vi "make_filename.vi"(8 "error in (no error)":errorcluster, 10 "Storage parameters":T1, 11 "Fileno.":i32) -> (0 "error out":errorcluster, 3 "Path":path)   [LabVIEW 2010]
uses:
  typedefs/storage_parameters_cluster.ctl
panel:
  # "_0000.txt"
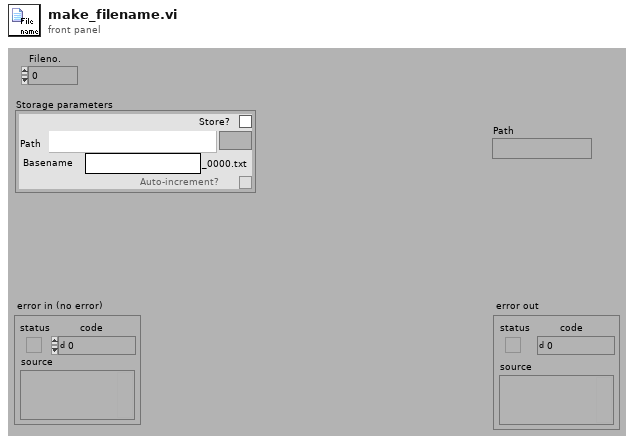
[diagram p1: front panel]
types:
  T1 = typedef "storage_parameters_cluster.ctl" = cluster{"Store?":bool, "Path":path, "Basename":string, "Auto-increment?":bool}
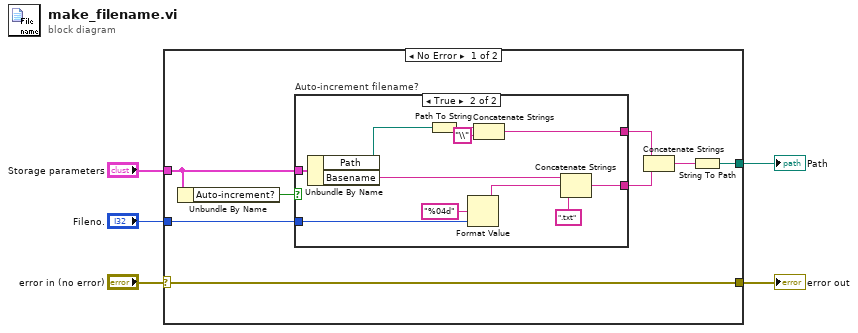
[diagram p0: block diagram]
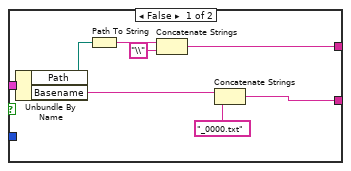
[diagram p2: hidden frame]
diagram:
  n1 = case shown="No Error" "error in (no error)" {
    selector: "error in (no error)" -> [w9 w33]
    tunnel: [w9 w33] -> w4
    tunnel: "Storage parameters" -> [w7 _]
    tunnel: "Fileno." -> [w13 _]
    tunnel: [w8 _] -> w1
    frame No Error {
      n2 = Unbundle By Name(w7) -> ("Auto-increment?"=w6:bool)
      n3 = case "Auto-increment filename?" shown="True" w6 {
        tunnel: w7 -> [w21 w32]
        tunnel: w13 -> [_ w26]
        tunnel: [w16 w28] -> w12
        tunnel: [w17 w27] -> w11
        frame False {
          n4 = Unbundle By Name(w21) -> ("Path"=w20:path, "Basename"=w15:string)
          n5 = Path To String(path=w20) -> (string=w19:string)
          n6 = Concatenate Strings(w19, "\\" ("string")) -> (w17:string)
          n7 = Concatenate Strings(w15, "_0000.txt" ("string")) -> (w16:string)
        }
        frame True {
          n8 = Unbundle By Name(w32) -> ("Path"=w31:path, "Basename"=w23:string)
          n9 = Path To String(path=w31) -> (string=w30:string)
          n10 = Format Value(format string="%04d", value (0)=w26) -> (output string=w24:string)  [unwired: 1 in]
          n11 = Concatenate Strings(w30, "\\" ("string")) -> (w27:string)
          n12 = Concatenate Strings(w23, w24, ".txt" ("string")) -> (w28:string)
        }
      }
      n13 = Concatenate Strings(w11, w12) -> (w10:string)
      n14 = String To Path(string=w10) -> (path=w8:path)
    }
    frame Error {
    }
  }
  "error out" <- w4
  "Path" <- w1
